vi "Test Control Parameters.vi"() -> ()   [LabVIEW 2022 SP3]
uses:
  <vilib>/MakerHub/LINX/Public/Peripherals/PWM/PWM Set Duty Cycle 1 Chan.vi
  <vilib>/MakerHub/LINX/Public/Peripherals/Analog/Analog Read 1 Chan.vi
  <vilib>/MakerHub/LINX/Public/Peripherals/Analog/Analog Read N Chans.vi
  <vilib>/MakerHub/LINX/Private/Local IO/LinxAnalogRead.vi
  <vilib>/MakerHub/LINX/Public/Utilities/Check Channel.vi
  <vilib>/MakerHub/LINX/Public/Utilities/Open Serial.vi
  <vilib>/MakerHub/LINX/Public/Peripherals/PWM/PWM Set Duty Cycle N Chans.vi
  <vilib>/MakerHub/LINX/Private/Utilties/Generate Error.vi
  <vilib>/MakerHub/LINX/LMH-LINX.lvlib
panel:
  in  "Stop Button":bool
  out "Temperature Chart":dbl(graph)
  out "Temperature [Deg C]":dbl format="%#.1g"
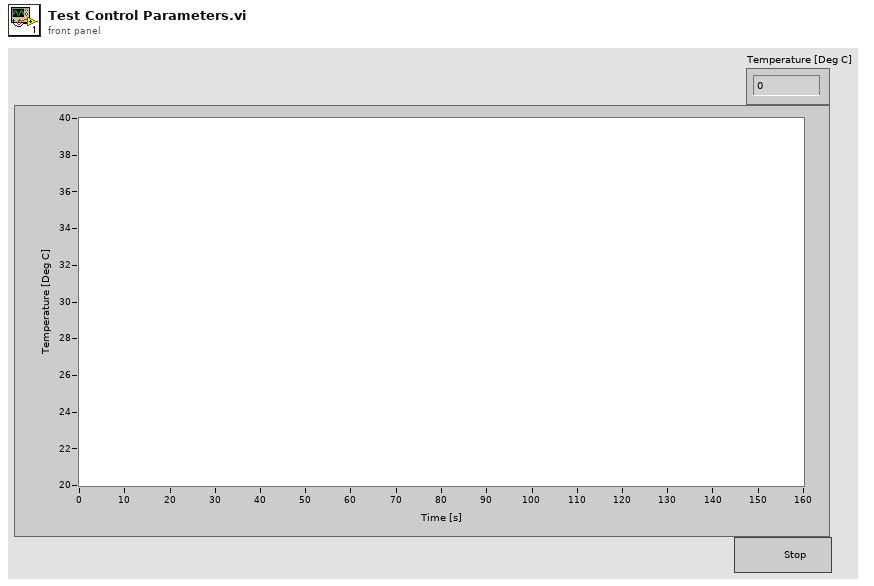
[diagram p1: front panel]
types:
  T1 = typedef "LMH-LINX.lvlib/LINX Ref.ctl" = cluster{"IO":T2, "Interface":T3, "LINX Device Config":T4}
  T2 = typedef "LMH-LINX.lvlib/Platform.ctl" = enum16{"Remote", "Local"}
  T3 = typedef "LMH-LINX.lvlib/Interface.ctl" = enum16{"Serial", "TCP"}
  T4 = typedef "LMH-LINX.lvlib/Device.lvlib/LINX Device Config.ctl" = cluster{"Interface":T3, "COM Port":refnum<visa-resource-name>, "TCP Configuration":T5, "Device Family":u8, "Device ID":u8, "Device Name":string, "TCP Ref":refnum<k5>, "Channels":T6}
  T5 = typedef "LMH-LINX.lvlib/Device.lvlib/TCP Config.ctl" = cluster{"IP Address":string, "Port":u16}
  T6 = typedef "LMH-LINX.lvlib/Channels.ctl" = cluster{"DI":u8[], "DO":u8[], "AI":u8[], "AO":u8[], "PWM":u8[], "QE":u8[], "UART":u8[], "I2C 2":u8[], "SPI":u8[], "CAN":u8[], "Servo":u8[], "AI Ref (V)":dbl, "AI Resolution (Bits)":u8, "AO Ref (V)":dbl, "AO Resolution (Bits)":u8}
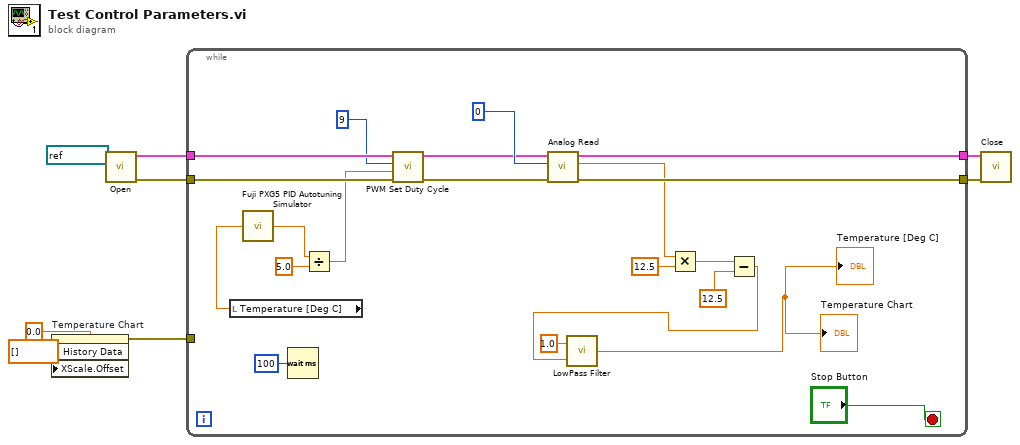
[diagram p0: block diagram]
diagram:
  n1 = property on="Temperature Chart" class="WFChart (strict)"("History Data"=dbl[] [], "XScale.Offset"=0.0 ("X Scale.Offset and Multiplier:Offset")) -> (error out=w1:errorcluster)  [unwired: 2 in, 1 out]
  n2 = call-poly <vilib>:"Open.vi"("Serial Port"=refnum<visa-resource-name> "COM8") -> ("Error Out"=w8:errorcluster, "LINX Resource"=w6:T1)  [unwired: 8 in, 1 out]
  n3 = while {
    tunnel: w8 -> [w25]
    tunnel: [w29] -> w7
    tunnel: w6 -> [w22]
    tunnel: [w28] -> w5
    tunnel: w1 -> [_]
    stop <- "Stop Button" stop-if-true
    n4 = local read "Temperature [Deg C]"() -> (w9:dbl)
    n5 = call "Fuji PXG5 PID Autotuning Simulator.vi"("PV [°C]"=w9) -> ("MV [V]"=w10:dbl)
    n6 = Wait (ms)(milliseconds to wait=u32 100) -> ()  [unwired: 1 out]
    n7 = Divide(x=w10, y=5.0) -> (x/y=w19:dbl)
    n8 = call-poly <vilib>:"PWM Set Duty Cycle.vi"("Error In"=w25, "Duty Cycle (0-1)"=w19, "PWM Channel"=u8 9 ("AO Channel"), "LINX Resource"=w22) -> ("Error Out"=w24:errorcluster, "LINX Resource"=w23:T1)  [unwired: 6 in]
    n9 = call-poly <vilib>:"Analog Read.vi"("Error In"=w24, "Analog Channel"=u8 0, "LINX Resource"=w23) -> ("Error Out"=w29:errorcluster, "Voltage"=w15:dbl, "LINX Resource"=w28:T1)  [unwired: 5 in, 1 out]
    n10 = Multiply(x=w15, y=12.5) -> (x*y=w17:dbl)
    n11 = Subtract(x=w17, y=12.5) -> (x-y=w11:dbl)
    n12 = call "LowPass Filter.vi"("Filter Input"=w11, "Ts [s]"=1.0) -> ("Filter Output"=→"Temperature [Deg C]" →"Temperature Chart":dbl)
  }
  n13 = call <vilib>:"Close.vi"("Error In"=w7, "LINX Resource"=w5) -> ()  [unwired: 9 in, 1 out]
